vi "set_setpoint_one.vi"(8 "error in (no error)":errorcluster, 10 "Setpoint temperature (instr units)":dbl min=-10.0 max=80.0 step=0.1 format="%#.1f", 11 "VISA resource name":refnum<visa-resource-name>) -> (0 "error out":errorcluster, 1 "Unit":string, 2 "Temperature":dbl, 3 "VISA resource name out":refnum<visa-resource-name>)   [LabVIEW 2018]
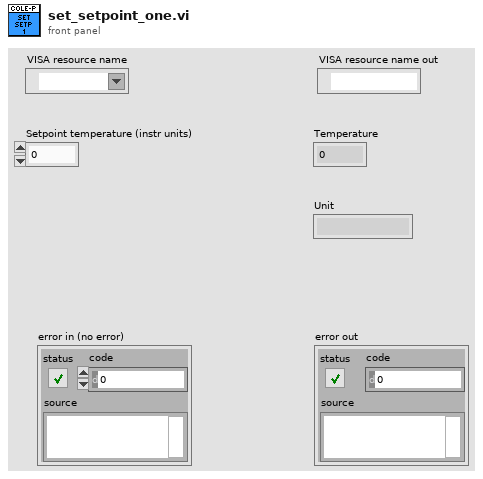
[diagram p1: front panel]
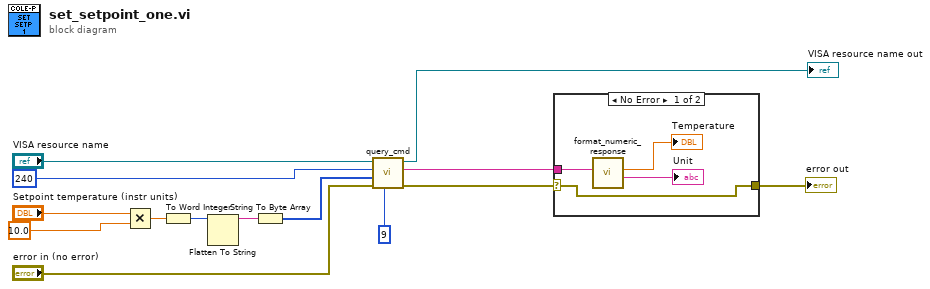
[diagram p0: block diagram]
diagram:
  n1 = Multiply(x="Setpoint temperature (instr units)", y=10.0) -> (x*y=w4:dbl)
  n2 = To Word Integer(number=w4) -> (16bit integer=w3:i16)
  n3 = Flatten To String(anything=w3) -> (data string=w2:string)  [unwired: 3 in, 2 out]
  n4 = String To Byte Array(string=w2) -> (unsigned byte array=w1:u8[])
  n5 = call "query_cmd.vi"("Number of bytes in response"=u32 9, "error in (no error)"="error in (no error)", "Data bytes"=w1, "Command byte"=u8 240, "VISA resource name"="VISA resource name") -> ("error out"=w8:errorcluster, "Response"=w9:string, "VISA resource name out"=→"VISA resource name out":refnum<visa-resource-name>)  [unwired: 4 in]
  n6 = case shown="No Error" w8 {
    selector: w8 -> [w15 w19]
    tunnel: w9 -> [w18 _]
    tunnel: [w15 w19] -> w7
    frame No Error {
      n7 = call "format_numeric_response.vi"("Response"=w18) -> ("Unit"=→"Unit":string, "Value"=→"Temperature":dbl)  [unwired: 9 in]
    }
    frame Error {
    }
  }
  "error out" <- w7
